vi "Read General Settings.vi"(8 "error in":errorcluster) -> (0 "error out":errorcluster, 2 "General":T1)   [LabVIEW 2011, in "GraphicalTestRunner.lvlib"]
uses:
  GraphicalTestRunner.lvlib
  <vilib>/Utility/config.llb/NI_LVConfig.lvlib
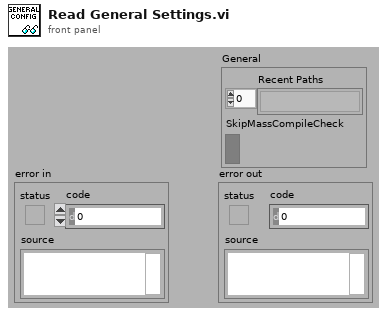
[diagram p1: front panel]
types:
  T1 = cluster{"Recent Paths":path[], "SkipMassCompileCheck":bool}
  T2 = typedef "NI_LVConfig.lvlib/Config Data RefNum.ctl" = refnum<k1>
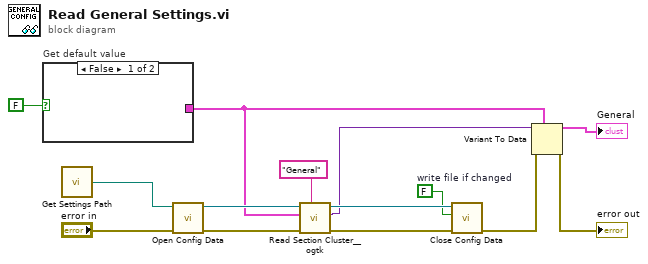
[diagram p0: block diagram]
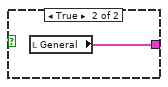
[diagram p2: hidden frame]
diagram:
  w8 = FALSE  # write file if changed
  n1 = case "Get default value" shown="False" FALSE {
    tunnel: [_ w15] -> w5
    frame False {
    }
    frame True {
      n2 = local read "General"() -> (w15:T1)
    }
  }
  n3 = call "Get Settings Path.vi"() -> ("config path"=w9:path)
  n4 = call <vilib>:"Open Config Data.vi"("error in (no error)"="error in", "configuration file path"=w9) -> ("error out"=w13:errorcluster, "refnum"=w11:T2)  [unwired: 7 in, 1 out]
  n5 = call <userlib>:"Read Section Cluster__ogtk.vi"("section (optional)"="General", "error in (no error)"=w13, "Section Formatted Cluster Type"=w5, "refnum"=w11) -> ("error out"=w12:errorcluster, "Section Formatted Cluster"=w7:variant, "dup refnum"=w10:T2)  [unwired: 3 in, 2 out]
  n6 = call <vilib>:"Close Config Data.vi"("error in (no error)"=w12, "write file if changed (T)"=w8, "refnum"=w10) -> ("error out"=w3:errorcluster)  [unwired: 7 in, 1 out]
  n7 = Variant To Data(error in=w3, type=w5, Variant=w7) -> (data=→"General":T1, error out=→"error out":errorcluster)
